vi "Get_KPRO_data_from_file 2016.vi"(11 "Output File KPRO Test":path=path "c:/KPRO_001.txt") -> (0 "Last_height_of_box":dbl format="%.2f", 1 "Last_depth_to_water":dbl format="%.2f", 2 "Last_depth":dbl format="%.2f", 3 "Output_array":sgl[][](array[numeric]) format="%.2f")   [LabVIEW 2016]
uses:
  <vilib>/Utility/file.llb/Read Delimited Spreadsheet (string).vi
  <vilib>/Utility/file.llb/Read Delimited Spreadsheet (DBL).vi
panel:
  out "first row":string[](array[string])
  out "report_header_length":i32
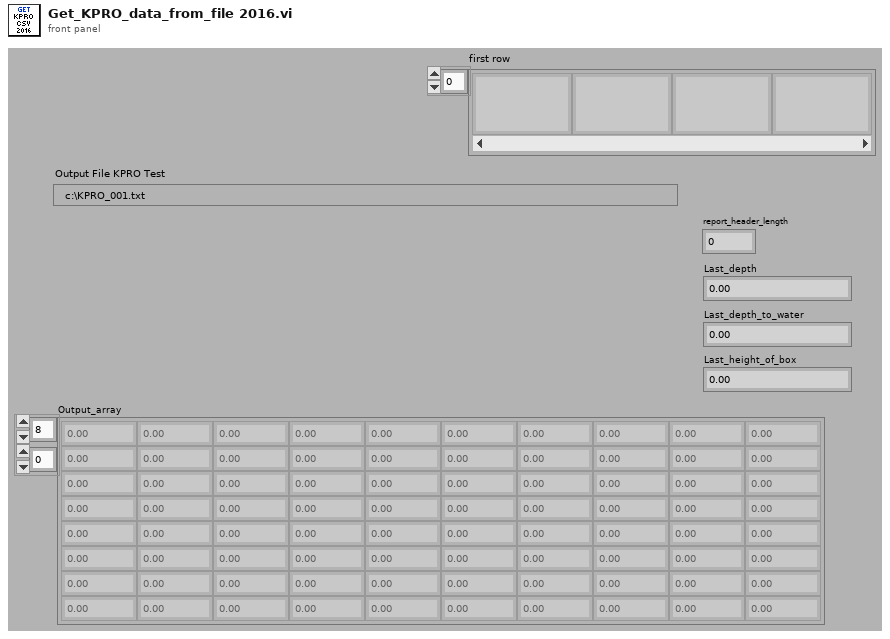
[diagram p1: front panel]
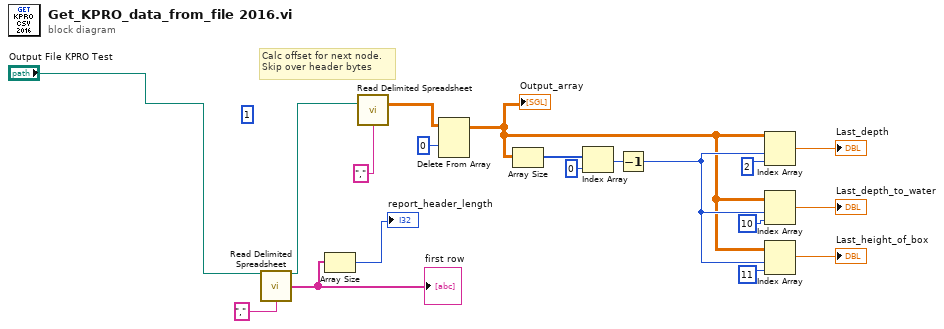
[diagram p0: block diagram]
diagram:
  (unwired) 1 ("number of lines (all:-1)")
  # "Calc offset for next node.\nSkip over header bytes"
  n1 = call-poly <vilib>:"Read Delimited Spreadsheet.vi"("file path (dialog if empty)"="Output File KPRO Test", "delimiter (\\t)"="," ("delimiter (\\t)")) -> ("new file path (Not A Path if cancelled)"=w7:path, "first row"=w6:string[])  [unwired: 8 in, 4 out]
  "first row" <- w6
  n2 = Array Size(array=w6) -> (size(s)=→"report_header_length":i32)
  n3 = call-poly <vilib>:"Read Delimited Spreadsheet.vi"("file path (dialog if empty)"=w7, "delimiter (\\t)"="," ("delimiter (\\t)")) -> ("all rows"=w4:dbl[][])  [unwired: 8 in, 5 out]
  n4 = Delete From Array(array=w4, index (row)=0) -> (array with subset deleted=w3:dbl[][])  [unwired: 2 in, 1 out]
  "Output_array" <- w3
  n5 = Array Size(array=w3) -> (size(s)=w18:i32[])
  n6 = Index Array(array=w18, index=0) -> (element=w16:i32)
  n7 = Decrement(x=w16) -> (x-1=w14:i32)
  n8 = Index Array(array=w3, index (row)=w14, index (col)=2 ("index")) -> (element=→"Last_depth":dbl)
  n9 = Index Array(array=w3, index (row)=w14, index (col)=10 ("disabled index (col)")) -> (element=→"Last_depth_to_water":dbl)
  n10 = Index Array(array=w3, index (row)=w14, index (col)=11 ("index")) -> (element=→"Last_height_of_box":dbl)
